vi "DAQmx_settings_update.vi"(0 "Task in":refnum<k21>, 1 "?":T1={"maximum value"=8.0, "minimum value"=-5.0, "samples per channel"=100, "Sample rate"=1000.0, "physical channels"="Dev1/ai0", "sample mode"=10123, "Itterations"=0, "source"="OnboardClock"} {"sample mode" items=["Finite Samples"=10178, "Continuous Samples"=10123, "Hardware Timed Single Point"=12522]; "Sample rate" format="%0.2f"; "minimum value" format="%0.2f"; "maximum value" format="%0.2f"}, 3 "error in":errorcluster) -> (7 "Task out":refnum<k21>, 10 "error out":errorcluster)   [LabVIEW 2020]
uses:
  controls/DAQmx_settings.ctl
  <resource>/objmgr/daqmx.rc
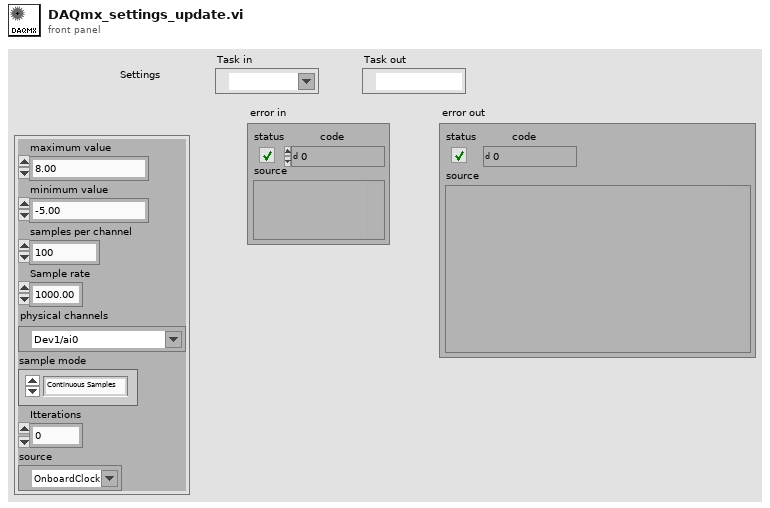
[diagram p1: front panel]
types:
  T1 = typedef "DAQmx_settings.ctl" = cluster{"maximum value":dbl, "minimum value":dbl, "samples per channel":i32, "Sample rate":dbl, "physical channels":tag, "sample mode":i32, "Itterations":u16, "source":tag}
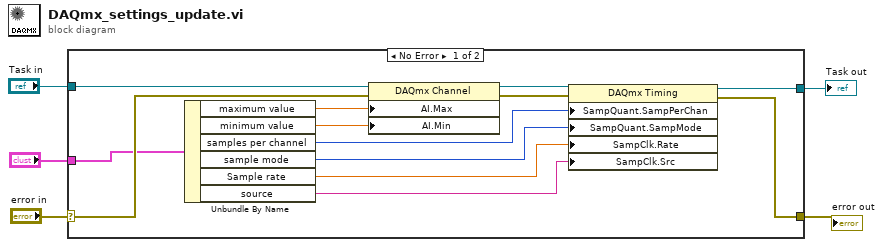
[diagram p0: block diagram]
diagram:
  n1 = case shown="No Error" "error in" {
    selector: "error in" -> [w18 w20]
    tunnel: [w16 w20] -> w4
    tunnel: "?" -> [w12 _]
    tunnel: "Task in" -> [w14 w19]
    tunnel: [w13 w19] -> w1
    frame No Error {
      n2 = Unbundle By Name(w12) -> ("maximum value"=w11:dbl, "minimum value"=w10:dbl, "samples per channel"=w9:i32, "sample mode"=w8:i32, "Sample rate"=w7:dbl, "source"=w6:tag)
      n3 = property class="DAQmx Channel"(reference=w14, error in=w18, "AI.Max"=w11, "AI.Min"=w10) -> (reference out=w15:refnum<k21>, error out=w17:errorcluster)
      n4 = property class="DAQmx Timing"(reference=w15, error in=w17, "SampQuant.SampPerChan"=w9, "SampQuant.SampMode"=w8, "SampClk.Rate"=w7, "SampClk.Src"=w6) -> (reference out=w13:refnum<k21>, error out=w16:errorcluster)
    }
    frame Error {
    }
  }
  "error out" <- w4
  "Task out" <- w1
